vi "Get All Timestamps.vi"(11 "Bytes in":u8[](array[numeric])) -> (1 "First and Last Timestamps":T1, 2 "Timestamps":i64[](array[numeric]), 3 "Bytes out":u8[](array[numeric]), 4 "Offsets":i32[](array[numeric]))   [LabVIEW 2021, in "pcap_Parse_Build_CIF.lvclass"]
doc: "Get all timestamps from pcap bytestream. This will automatically detect if a global header is present and will work on both full pcap streams to/from disk and pcap packets to/from FIFO."
uses:
  pcap_Parse_Build_CIF.lvclass
  Typedef/First and Last Timestamps.ctl
  pcap_Parse_Build_CIF.lvclass/pcap_Parse_Build_CIF.ctl
  Add Error.vi
  Parse/Unflatten Packet Header.vi
  <vilib>/CIF Foundation/CIF Utilities/Errors/Append Error Location.vi
  <vilib>/CIF Foundation/CIF Utilities/DataTypes/Flatten Unflatten/Unflatten U32.vi
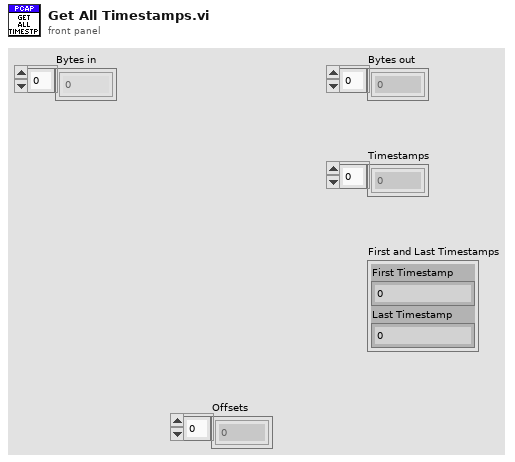
[diagram p1: front panel]
types:
  T1 = typedef "pcap_Parse_Build_CIF.lvclass/First and Last Timestamps.ctl" = cluster{"First Timestamp":i64, "Last Timestamp":i64}
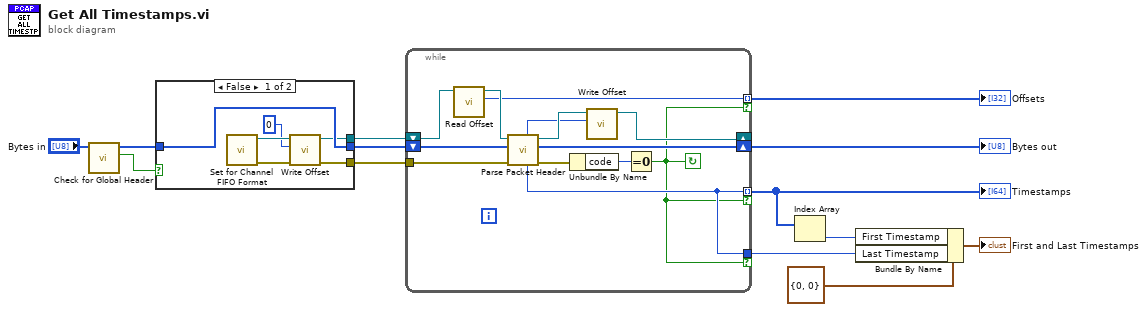
[diagram p0: block diagram]
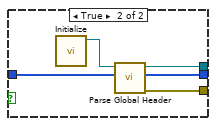
[diagram p2: hidden frame]
diagram:
  n1 = call "Check for Global Header.vi"("Bytes in"="Bytes in") -> ("Global Header Present"=w13:bool, "Bytes out"=w10:u8[])  [unwired: 8 in, 1 out]
  n2 = case shown="False" w13 {
    tunnel: [w15 w20] -> w9
    tunnel: w10 -> [w17 w23]
    tunnel: [w17 w22] -> w12
    tunnel: [w18 w21] -> w11
    frame False {
      n3 = call "Set for Channel FIFO Format.vi"() -> ("error out"=w18:errorcluster, "pcap_Parse_Build_CIF out"=w16:refnum<class "pcap_Parse_Build_CIF.lvclass">)  [unwired: 10 in]
      n4 = call "Write Offset.vi"("Offset"=0, "pcap Parse and Build in"=w16) -> ("pcap Parse and Build out"=w15:refnum<class "pcap_Parse_Build_CIF.lvclass">)  [unwired: 8 in, 1 out]
    }
    frame True {
      n5 = call "Initialize.vi"() -> ("pcap Parse and Build out"=w19:refnum<class "pcap_Parse_Build_CIF.lvclass">)  [unwired: 11 in]
      n6 = call "Parse Global Header.vi"("Bytes in"=w23, "pcap Parse and Build in"=w19) -> ("error out"=w21:errorcluster, "Bytes out"=w22:u8[], "pcap Parse and Build out"=w20:refnum<class "pcap_Parse_Build_CIF.lvclass">)  [unwired: 6 in, 1 out]
    }
  }
  n7 = while {
    tunnel: w11 -> [w35]
    shift-right: [w33] -> _
    shift-left: w9 -> [w27]
    tunnel: [w28] -> w6 mode=indexing if=w24
    shift-right: [w29] -> w7
    shift-left: w12 -> [w36]
    tunnel: [w28] -> w3 if=w24
    tunnel: [w25] -> w1 mode=indexing if=w24
    stop <- w24 continue-if-true
    n8 = call "Read Offset.vi"("pcap Parse and Build in"=w27) -> ("Offset"=w25:i32, "pcap Parse and Build out"=w26:refnum<class "pcap_Parse_Build_CIF.lvclass">)  [unwired: 8 in, 1 out]
    n9 = call "Parse Packet Header.vi"("error in (no error)"=w35, "Bytes in"=w36, "pcap Parse and Build in"=w26) -> ("error out"=w31:errorcluster, "Bytes out"=w29:u8[], "pcap Parse and Build out"=w34:refnum<class "pcap_Parse_Build_CIF.lvclass">, "TAI Time (ns)"=w28:i64, "Next Packet offset"=w32:i32)  [unwired: 3 in, 1 out]
    n10 = Unbundle By Name(w31) -> ("code"=w30:i32)
    n11 = call "Write Offset.vi"("Offset"=w32, "pcap Parse and Build in"=w34) -> ("pcap Parse and Build out"=w33:refnum<class "pcap_Parse_Build_CIF.lvclass">)  [unwired: 8 in, 1 out]
    n12 = Equal To 0?(x=w30) -> (x = 0?=w24:bool)
  }
  "Timestamps" <- w6
  "Bytes out" <- w7
  "Offsets" <- w1
  n13 = Index Array(array=w6) -> (element=w4:i64)  [unwired: 1 in]
  n14 = Bundle By Name(cluster=T1 {"First Timestamp"=0, "Last Timestamp"=0} ("Timestamps (ns)"), "First Timestamp"=w4, "Last Timestamp"=w3) -> (→"First and Last Timestamps":T1)
